vi "SubPanel_DataCollection_Rev11_v15.vi"(0 "DCPowerInformationClusterArray_Input":T4(array[cluster]), 1 "VISAPowerInfoInputArray":T3(array[cluster]), 2 "Run Data SubPanel Input":T2, 3 "RF Block Input Array":T1[](array[typedef]), 4 "Oscilloscope Info Array":T7(array[cluster]) {"vertical coupling" items=["AC", "DC", "Ground"]}, 5 "Plot Color Array":u32[](array[colorbox])=[16711686, 65351, 8978420, 14474240, 16139007, 16752640, 8958719, 16758973, 16777215, 46792, 11992992, 12961221, 16763690, 12600063, 16711835, 2953983, 40796, 13111296, 13352613, 9221011, 12964076, 12819897, 65442, 16776704, 14540253, 16740729, 10658047, 10813344, 16753521, 13413843, 8691115, 10339240, 14401205, 16746704, 7467519, 16775978, 13872558, 11387603, 13354405, 10420227, 13107364, 4060, 35208, 11817216, 7566080, 40796, 7539456, 2837073, 6372186, 7499083, 10648702, 16757152], 6 "New Run?":bool, 7 "error in":errorcluster) -> (20 "DCPowerInformationClusterArray_Output":T4(array[cluster]), 21 "VISAPowerInfoInputOutput":T3(array[cluster]), 22 "Run Data SubPanel Output":T2, 23 "RF Subpanel Output":T1[](array[typedef]), 24 "Oscilloscope Info Array":T7(array[cluster]) {"vertical coupling" items=["AC", "DC", "Ground"]}, 25 "Reinitialize?":bool, 26 "Data Was Collected?":bool, 27 "error out":errorcluster)   [LabVIEW 2019]
uses:
  Controls/DataBlockControl.ctl
  Controls/QueueDataControl_V3.ctl
  <vilib>/Utility/file.llb/Write Delimited Spreadsheet (string).vi
  <instrlib>/niScope/Acquire/Fetch/niScope Multi Fetch Binary 16.vi
  Controls/RFBlockControl.ctl
  <instrlib>/niScope/Controls/niScope vertical coupling.ctl
panel:
  in  "Total Current Y Min":dbl
  in  "Total Current Y Max":dbl
  in  "Total Voltage Y Min":dbl
  in  "Total Voltage Y Max":dbl
  in  "Total Measurement Range Update":bool
  in  "Live Measurement Range Update":bool
  in  "Live Current Y Min":dbl
  in  "Live Current Y Max":dbl
  in  "Live Voltage Y Min":dbl
  in  "Live Voltage Y Max":dbl
  out "Current Measurements Live":cluster{dbl[], dbl[]}[](graph)
  out "Voltage Measurements Live":cluster{dbl[], dbl[]}[](graph)
  out "RFSourceInfoArray":string[][](array[string])
  out "OscilloscopeInfoArray":string[][](array[string])
  out "Voltage Waveform Array":waveform(dbl)[](graph)
  out "Current Waveform Array":waveform(dbl)[](graph)
  out "DCPowerInfoArray":string[][](array[string])
  out "Current Measurements Total":cluster{dbl[], dbl[]}[](graph)
  out "Voltage Measurements Total":cluster{dbl[], dbl[]}[](graph)
  out "Exiting":bool
  out "Full Run Information":string
  out "Ready For Next Run?":bool
  in  "Next Run":bool
  out "Recording Data":bool
  in  "Record Data Toggle":bool
  out "error of collection":errorcluster
  in  "force exit SubVI":bool
  out "RF Block Parameters Output":T1
  in  "Oscilloscope Info Array":T6(array[cluster]) {"vertical coupling" items=["AC", "DC", "Ground"]}
  # "Background information (Important)\nThere are three sets of voltage/current graphs\n\nOne is live always and just shows what all the channels look like _______ Waveform Array\n\nOne is live when measuring and shows some duration of the recording _______ Measurements Live\n\nOne shows the entire duration of the run, but it will take a few seconds to compile, just be patient it will populate\n\n\nInstructions (More Important)"
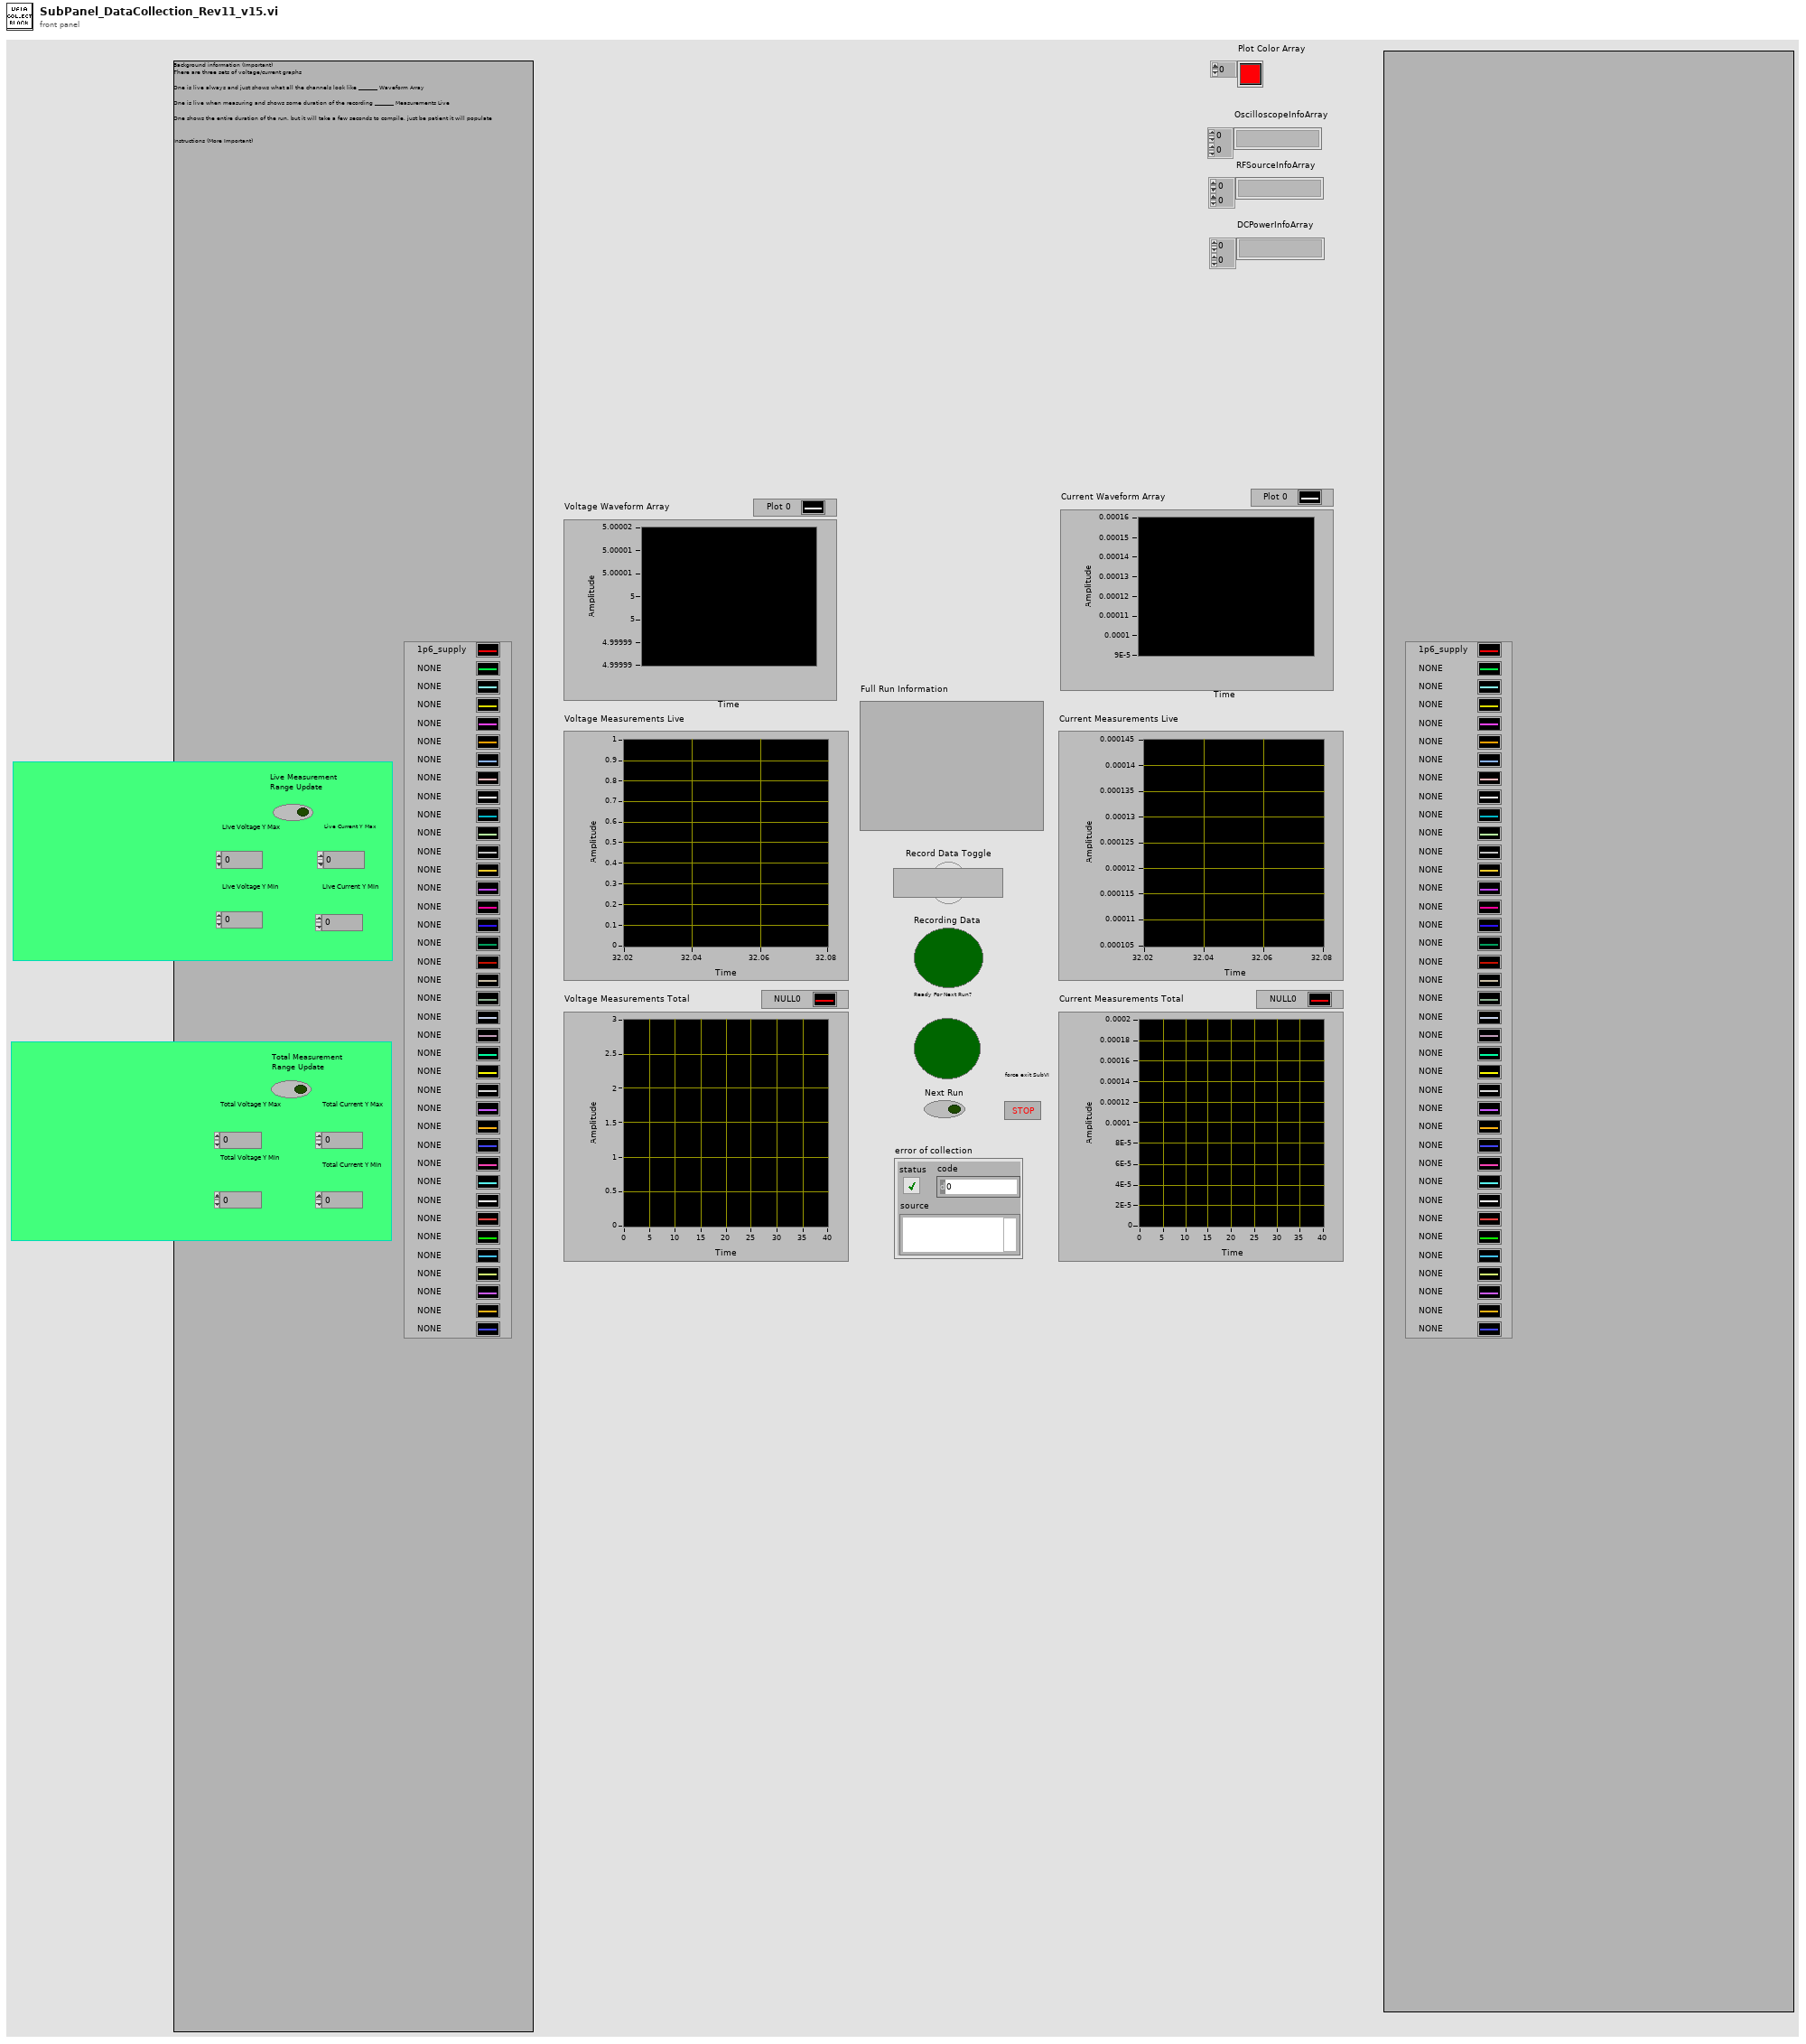
[diagram p1: front panel]
types:
  T1 = typedef "RFBlockControl.ctl" = cluster{"VISA resource name":refnum<visa-resource-name>, "RF Power State In":bool, "Frequency (GHz) Output":dbl, "Power (dBm) Output":dbl, "Instrument Name":string}
  T2 = typedef "DataBlockControl.ctl" = cluster{"Run Folder Parent Directory":path, "DUT":string, "Ion (ex Kr)":string, "Board Number":string, "Effective LET":string, "Test Type":enum16{"Single Event Latchup", "Single Event Transient", "Single Event Upset"}}
  T3 = cluster{"VISA resource name":refnum<visa-resource-name>, "String List":string, string[], "Input Array (Voltage,Current_Limit)":dbl[], "Input Array (Voltage,Current_Limit)":dbl[], "Channel Names":string[], "read buffer":string}[]
  T4 = cluster{"instrument handle out":refnum<k15>, string, string[], dbl[], string[], "Current Limit Output Array":dbl[], dbl[]}[]
  T5 = typedef "niScope vertical coupling.ctl" = i32
  T6 = cluster{"instrument handle out":refnum<k15>, "channel numbers array":string[], "channel names array":string[], "vertical range":dbl, "vertical coupling":T5, "Channel 0 50 ohms?":bool, "50 ohm vertical range (V)":dbl, "min record length":i32, "Actual Sample Rate":dbl}[]
  T7 = cluster{"instrument handle out":refnum<k15>, string[], string[], "vertical range":dbl, "vertical coupling":T5, "Channel 0 50 ohms?":bool, "50 ohm vertical range (V)":dbl, "min record length":i32, "Actual Sample Rate":dbl, "channel names list":string}[]
  T8 = typedef "QueueDataControl_V3.ctl" = cluster{"Array of fetched data":dbl[][][], "Channel Names Array":string[], "Voltage Waveform Array":waveform(dbl)[], "Current Waveform Array":waveform(dbl)[], "Resetting Time":timestamp, "Beam Logic":dbl}
  T9 = cluster{"IVI Refnum out":refnum<k15>, string, "voltage level channel 23":dbl, "Channel Name 23":string, "Current Limit":dbl, "Measure Record dt":dbl, string}[]
  T10 = cluster{timestamp[], "wfm info":cluster{"actualSamples":i32, "absoluteInitialX":dbl, "relativeInitialX":dbl, "xIncrement":dbl, "offset":dbl, "gain":dbl, "reserved1":dbl, "reserved2":dbl}[][], "wfm":i16[][][]}
  T11 = cluster{"actualSamples":i32, "absoluteInitialX":dbl, "relativeInitialX":dbl, "xIncrement":dbl, "offset":dbl, "gain":dbl, "reserved1":dbl, "reserved2":dbl}[]
  T12 = cluster{"created path array":path[], "DCPowerInformation_byChannel":cluster{"IVI Refnum out":refnum<k15>, string, "voltage level channel 23":dbl, "Channel Name 23":string, "Current Limit":dbl, "Measure Record dt":dbl, string}[], string[]}
  T13 = cluster{"Array of fetched data":dbl[][], string, i32[]}
  T14 = enum16{"open", "replace", "create", "open or create", "replace or create", "replace or create with confirmation"}
  T15 = enum16{"Single Event Latchup", "Single Event Transient", "Single Event Upset"}
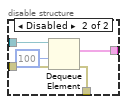
[diagram p6: hidden frame]
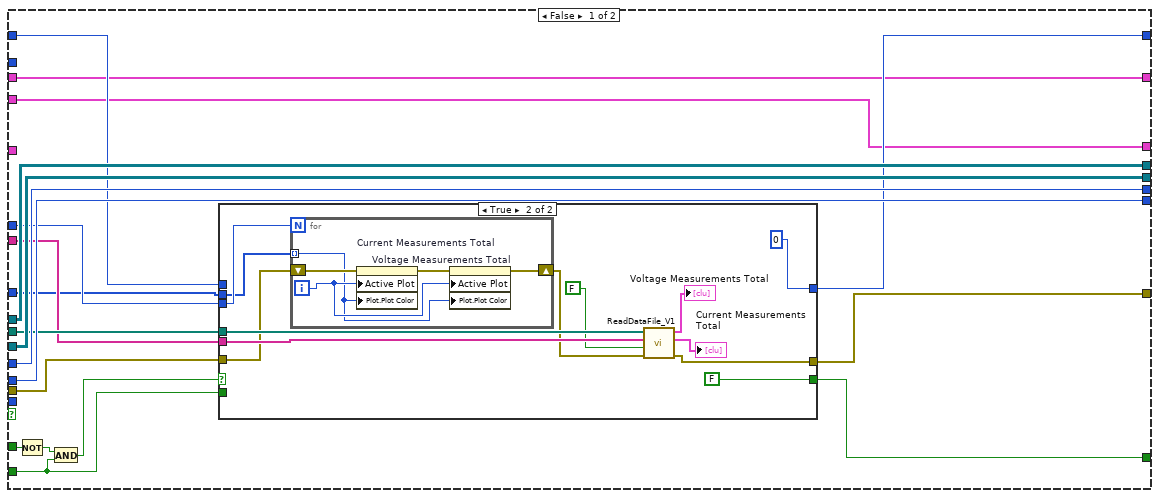
[diagram p7: hidden frame]
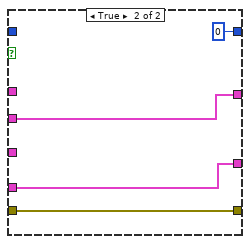
[diagram p9: hidden frame]
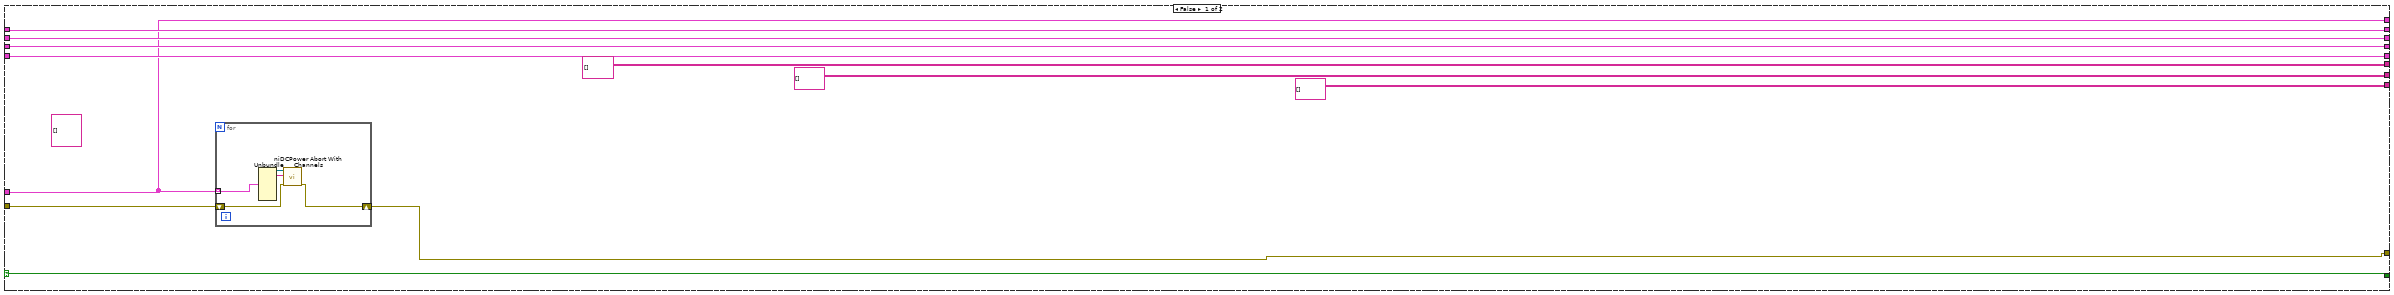
[diagram p10: hidden frame]
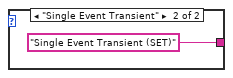
[diagram p11: hidden frame]
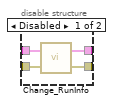
[diagram p15: hidden frame]
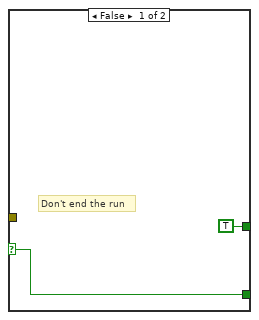
[diagram p18: hidden frame]
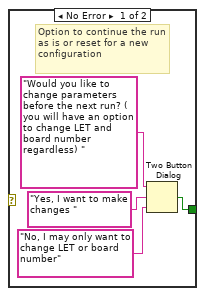
[diagram p19: hidden frame]
diagram:
  w18 = cluster{dbl[], dbl[]}[] [] ("array")
  (unwired) string[] ["Instrument Name", "Channel Name", "Instrument Channel Number", "Voltage (V)", "Current Limit (A)", "Measure Record delta Time (s)"] ("new element/subarray")
  w51 = T8 {"Array of fetched data"=[], "Channel Names Array"=[], "Voltage Waveform Array"=[], "Current Waveform Array"=[], "Resetting Time"=timestamp(0 s since 1904-01-01), "Beam Logic"=0.0} ("DCPower Queue Data Double Array Format")
  (unwired) T8 {"Array of fetched data"=[], "Channel Names Array"=[], "Voltage Waveform Array"=[], "Current Waveform Array"=[], "Resetting Time"=timestamp(0 s since 1904-01-01), "Beam Logic"=0.0} ("DCPower Double Array Queue")
  (unwired) 10000 ("binary file indexor in")
  (unwired) T2 {"Run Folder Parent Directory"=path "", "DUT"="", "Ion (ex Kr)"="", "Board Number"="", "Effective LET"="", "Test Type"=enum."Single Event Latchup"} ("Run Data Configuration")
  # "Need to make a function that will decrease the amount of loops if there are more channels active. Just exponential decay or a X/Y function but need some kind of offset which will probably be experimentally determined"
  # "Initiating the queue"
  # "echoing run information"
  # "Checking if this is a new run. If it is, a new folder is created along with references to a datafile node. If it is not new (i.e. you didn't start recording data because you needed to make a last minute change and pressed forced exit subvi), the previous folder that is theoretically empty (or just has the .txt files is used"
  # "If yes, you go into this subVI"
  # "This is the message at the beginning confirming if you want to make small changes to the program (i.e. LET)"
  # "Parameters from the configuration stage of this program"
  # "Reset the graph that is saving every 10 seconds of data. Every reset the low bound of the ten seconds is"
  # "Need to change to reflect number of channels that are being recorded. Collect this from a parameters file eventually that will be created"
  # "Indicator if the system is ready for another run. Also indicates if data was actually collected"
  # "Resets the system to start recording"
  # "A flag to ensure the warning message shows only once and doesn't lock the system"
  # "Initiating all of the DC Power instruments (doing this here so because we force abort channels in the DCPower setup because buffer overflow issues. Iterating over the instrument array and the active channel list"
  n1 = flat-sequence {
    tunnel: [w90] -> w67
    tunnel: "error in" -> [w80]
    tunnel: [w94] -> w72
    tunnel: "Run Data SubPanel Input" -> [w82]
    frame #0 {
      n2 = disable-structure shown="Enabled" {
        disable-tunnel: w80 -> [w97 w108]
        disable-tunnel: [w106 w108] -> w79
        frame Enabled {
          n3 = property on="Voltage Measurements Live" class="XYGraph (strict)"(error in=w97, "BG Color"=u32 0 ("Plot.Plot Color"), "Plot.Plot Interpolation"=u8 2) -> (error out=w96:errorcluster)  [unwired: 1 in, 1 out]
          n4 = property on="Current Measurements Live" class="XYGraph (strict)"(error in=w96, "BG Color"=u32 0 ("Plot.Plot Color"), "Plot.Plot Interpolation"=u8 2) -> (error out=w95:errorcluster)  [unwired: 1 in, 1 out]
          n5 = property on="Voltage Measurements Total" class="XYGraph (strict)"(error in=w95, "BG Color"=u32 0 ("Plot.Plot Color"), "Plot.Plot Interpolation"=u8 2) -> (error out=w107:errorcluster)  [unwired: 1 in, 1 out]
          n6 = property on="Current Measurements Total" class="XYGraph (strict)"(error in=w107, "BG Color"=u32 0 ("Plot.Plot Color"), "Plot.Plot Interpolation"=u8 2) -> (error out=w106:errorcluster)  [unwired: 1 in, 1 out]
        }
        frame Disabled {
        }
      }
      n7 = local write "Voltage Measurements Total"(cluster{dbl[], dbl[]}[] [] ("Voltage Measurements")) -> ()
      n8 = local write "Current Measurements Total"(cluster{dbl[], dbl[]}[] [] ("Current Measurements")) -> ()
      n9 = local write "Recording Data"(FALSE ("Recording Data")) -> ()
      n10 = local write "Exiting"(FALSE ("Forced Exit")) -> ()
      n11 = call "Convert_RunInfoCluster_2_RunInfoStringList.vi"("error in"=w79, "Run Number"="", "Run Data SubPanel Input"=w82) -> ("error output"=w83:errorcluster, "Run Data Output"=w84:string)
      n12 = call "Display Message to User"("error in (no error)"=w83, "Enable"=TRUE, "Message"=w84) -> ("error out"=w90:errorcluster)  [unwired: 7 in, 1 out]
      n13 = Two Button Dialog(message="Changing the LET?", 1:"No" ("F button name (\"Cancel\")"), 2:"Yes" ("T button name (\"OK\")")) -> (T button?=w94:bool)
    }
  }
  n14 = call "Convert_InstrumentReferenceArray_2_ChannelReferenceArray.vi"("error in (no error)"=w67, "DCPowerInformationClusterArray_Input"="DCPowerInformationClusterArray_Input") -> ("error out"=w66:errorcluster, "DCPowerInformation_byChannel"=w12:T9)
  n15 = case shown="True" w72 {
    tunnel: "Run Data SubPanel Input" -> [w110 w114]
    tunnel: [w110 w113] -> w26
    tunnel: [w109 w112] -> w68
    tunnel: w66 -> [w109 w111]
    frame False {
    }
    frame True {
      n16 = disable-structure shown="Enabled" {
        disable-tunnel: w114 -> [w118 w120]
        disable-tunnel: [w117 w119] -> w113
        disable-tunnel: [w116 w122] -> w112
        disable-tunnel: w111 -> [w115 w121]
        frame Disabled {
          n17 = call "Change_RunInfo.vi"("error in (no error)"=w115, "Run Data SubPanel in"=w118) -> ("error out"=w116:errorcluster, "Run Data SubPanel out"=w117:T2)
        }
        frame Enabled {
          n18 = call "Change_RunInfo_V2.vi"("error in (no error)"=w121, "Run Data SubPanel in"=w120) -> ("error out"=w122:errorcluster, "Run Data SubPanel out"=w119:T2)
        }
      }
    }
  }
  n19 = Unbundle(w26) -> ("Run Folder Parent Directory"=w69:path)  [unwired: 5 out]
  n20 = List Folder(path=w69, error in=w68) -> (folder names=w70:string[], error out=w54:errorcluster)  [unwired: 2 in, 2 out]
  n21 = Array Size(array=w70) -> (size(s)=w57:i32)
  n22 = case shown="True" "New Run?" {
    selector: "New Run?" -> [w124 w127]
    tunnel: [w125 w129] -> w58
    tunnel: w57 -> [w125 w128]
    tunnel: [w124 w127] -> w56
    tunnel: [w123 w126] -> w55
    tunnel: w54 -> [w123 w126]
    frame False {
    }
    frame True {
      n23 = Increment(x=w128) -> (x+1=w129:i32)
    }
  }
  n24 = Number To Decimal String(number=w58) -> (decimal integer string=w61:string)  [unwired: 1 in]
  n25 = Concatenate Strings("Run_", w61) -> (w25:string)
  n26 = Array Size(array=w12) -> (size(s)=w53:i32)
  n27 = call "InitialFileFolderCreation_V2.vi"("New Run?"=w56, "error in (no error)"=w55, "Run Number"=w25, "Subfolders&NumChannelsRecorded"=w53, "base path"=w69) -> ("error out"=w24:errorcluster, "SupplementalDataFileReferenceObjectArrayWsubfolders"=w64:refnum<file>[][], "DataFileReferenceObjectArrayWsubfolders"=w65:refnum<file>[][], "created path array"=w30:path[])  [unwired: 3 in]
  n28 = call "Convert_RunInfoCluster_2_RunInfoStringList.vi"("error in"=w24, "Run Number"=w25, "Run Data SubPanel Input"=w26) -> ("error output"=w23:errorcluster, "Run Data Output"=→"Full Run Information":string)
  n29 = for {
    shift-right: [w130] -> w9
    shift-left: w23 -> [w132]
    tunnel: "DCPowerInformationClusterArray_Input" -> [w134] mode=indexing
    n30 = Unbundle(w134) -> ("instrument handle out"=w131:refnum<k15>, w133:string)  [unwired: 5 out]
    n31 = call <instrlib>:"niDCPower Initiate With Channels.vi"("error in (no error)"=w132, "channel name"=w133, "instrument handle"=w131) -> ("error out"=w130:errorcluster)  [unwired: 7 in, 1 out]
  }
  n32 = for {
    shift-right: [w137] -> w10
    shift-left: w9 -> [w139]
    tunnel: "Plot Color Array" -> [_] mode=indexing
    i -> [w135]
    w136 = "NONE" ("Plot.Plot Name")
    n33 = property on="Current Measurements Live" class="XYGraph (strict)"(error in=w139, "Active Plot"=w135, "Plot.Plot Name"=w136) -> (error out=w138:errorcluster)  [unwired: 1 in, 1 out]
    n34 = property on="Voltage Measurements Live" class="XYGraph (strict)"(error in=w138, "Active Plot"=w135, "Plot.Plot Name"=w136) -> (error out=w137:errorcluster)  [unwired: 1 in, 1 out]
  }
  n35 = case shown="Error .." w10 {
    selector: w10 -> [w140 _]
    tunnel: [w140 w141] -> w4
    tunnel: w9 -> [_ w141]
    frame No Error {
    }
    frame Error {
    }
  }
  n36 = for {
    tunnel: w12 -> [w144] mode=indexing
    tunnel: [w147] -> w13 mode=indexing
    shift-right: [w143] -> w14
    shift-left: w4 -> [w146]
    tunnel: "Plot Color Array" -> [w142] mode=indexing
    i -> [w148]
    # "Creating Array of Channel Names"
    n37 = Unbundle(w144) -> ("Channel Name 23"=w147:string)  [unwired: 6 out]
    n38 = property on="Current Measurements Live" class="XYGraph (strict)"(error in=w146, "Active Plot"=w148, "Plot.Plot Name"=w147, "Plot.Plot Color"=w142) -> (error out=w145:errorcluster)  [unwired: 1 in, 1 out]
    n39 = property on="Voltage Measurements Live" class="XYGraph (strict)"(error in=w145, "Active Plot"=w148, "Plot.Plot Name"=w147, "Plot.Plot Color"=w142) -> (error out=w143:errorcluster)  [unwired: 1 in, 1 out]
  }
  n40 = disable-structure shown="Enabled" {
    disable-tunnel: w14 -> [w152 w154]
    disable-tunnel: [w151 w154] -> w3
    disable-tunnel: [w150 _] -> w15
    disable-tunnel: w51 -> [w149 _]
    frame Enabled {
      n41 = Obtain Queue(name (unnamed)="DCPowerQueue", element data type=w149, error in (no error)=w152) -> (queue out=w150:refnum<queue>, error out=w151:errorcluster)  [unwired: 2 in, 1 out]
    }
    frame Disabled {
    }
  }
  n42 = disable-structure shown="Disabled" {
    disable-tunnel: "Oscilloscope Info Array" -> [w160 _]
    disable-tunnel: w3 -> [w159 _]
    frame Disabled {
      w155 = T10 {[], "wfm info"=[], "wfm"=[]} ("output cluster")
      n43 = Obtain Queue(name (unnamed)="OscilloscopeDataQueue", element data type=w155, error in (no error)=w159) -> (queue out=w156:refnum<queue>, error out=w158:errorcluster)  [unwired: 2 in, 1 out]
      n44 = Unbundle() -> ()  [unwired: 1 in, 2 out]
      n45 = while {
        shift-right: _ -> [_]
        shift-left: w158 -> [w169]
        shift-right: [w164] -> _
        shift-left: w160 -> [w164]
        tunnel: w156 -> [w167]
        tunnel: w155 -> [w166]
        stop <- _ stop-if-true
        # "BASE OFF OF TAMU POWER SCRIPTS"
        n46 = for {
          tunnel: w164 -> [w188] mode=indexing
          shift-right: [w182] -> w165
          shift-left: w169 -> [w183]
          tunnel: [w181] -> w162 mode=indexing
          tunnel: [w180] -> w161 mode=indexing
          tunnel: [w179] -> w163 mode=indexing
          n47 = Unbundle By Name(w188) -> ("instrument handle out"=w187:refnum<k15>, "channel names list"=w185:string)
          n48 = Get Date/Time In Seconds() -> (seconds since 1Jan1904=w179:timestamp)
          n49 = call-poly <instrlib>:"niScope Fetch (poly).vi"("timeout"=0.0, "error in"=w183, "numSamples"=-1, "channels"=w185, "instrument handle"=w187) -> ("error out"=w182:errorcluster, "wfm"=w180:i16[][], "wfm info"=w181:T11)  [unwired: 3 in, 1 out]
        }
        n50 = Bundle(cluster=w166, w163, "wfm info"=w162, "wfm"=w161) -> (w168:T10)
        n51 = for {
          tunnel: w163 -> [w171] mode=indexing
          tunnel: w162 -> [w175]
          tunnel: w161 -> [w174]
          i -> [w173]
          n52 = Index Array(array=w175, index (col)=w173) -> (element=w172:T11)  [unwired: 1 in]
          n53 = Index Array(array=w174, index (dim 0)=w173) -> (element=w170:i16[][])  [unwired: 2 in]
          n54 = for {
            tunnel: w172 -> [w178] mode=indexing
            tunnel: w171 -> [w177]
            tunnel: w170 -> [_] mode=indexing
            n55 = Unbundle(w178) -> ("xIncrement"=w176:dbl)  [unwired: 7 out]
            n56 = Bundle By Name("dt"=w176, "t0"=w177) -> ()  [unwired: 2 in, 1 out]
          }
        }
        n57 = Enqueue Element(queue=w167, element=w168, error in (no error)=w165) -> ()  [unwired: 1 in, 3 out]
      }
      n58 = while {
        stop <- _ stop-if-true
      }
    }
    frame Enabled {
    }
  }
  n59 = Bundle("created path array"=w30, "DCPowerInformation_byChannel"=w12, w13) -> (w43:T12)  [unwired: 1 in]
  n60 = Array Size(array=w13) -> (size(s)=w17:i32)
  n61 = Get Date/Time In Seconds() -> (seconds since 1Jan1904=w28:timestamp)
  n62 = while {
    tunnel: w15 -> [w228]
    shift-right: [w189] -> w48
    shift-left: w3 -> [w227]
    tunnel: w30 -> [w224]
    shift-right: [w217] -> w50
    shift-left: w65 -> [w225]
    shift-right: [w216] -> w49
    shift-left: w64 -> [w223]
    shift-right: [w219] -> _
    shift-left: 0 ("binary file indexor in") -> [w222]
    shift-right: [w218] -> _
    shift-left: 0 ("binary file indexor in") -> [w221]
    tunnel: 1000 ("binary file indexor in") -> [w220]
    tunnel: w13 -> [w226]
    tunnel: w17 -> [w195]
    shift-right: [w205] -> _
    shift-left: FALSE -> [w204]
    shift-right: [w201] -> _
    shift-left: 0 -> [w202]
    shift-right: [w200] -> _
    shift-left: w18 -> [w197]
    shift-right: [w199] -> _
    shift-left: w18 -> [w198]
    tunnel: 251 ("y") -> [w196]
    tunnel: "Plot Color Array" -> [w194]
    stop <- w213 stop-if-true
    # "If recording data is on, there should always be elements in the queue, so I shouldn't have to worry about a state where the \"recording data\" is active but there is no data in the queue, if so, then I'll just have to find an alternative to the OR statement"
    n63 = Get Queue Status(queue=w228, error in (no error)=w227) -> (queue out=w210:refnum<queue>, error out=w211:errorcluster, # elements in queue=w206:i32)  [unwired: 1 in, 5 out]
    n64 = local read "Recording Data"() -> (w203:bool)
    n65 = disable-structure shown="Enabled" {
      disable-tunnel: [w248 w250] -> w212
      disable-tunnel: w211 -> [w247 w252]
      disable-tunnel: w210 -> [w246 w253]
      disable-tunnel: [w245 w249] -> w209
      frame Enabled {
        n66 = Flush Queue(queue=w246, error in (no error)=w247) -> (remaining elements=w245:T8[], error out=w248:errorcluster)  [unwired: 1 out]
      }
      frame Disabled {
        n67 = Dequeue Element(queue=w253, timeout in ms (-1)=100, error in (no error)=w252) -> (element=w249:T8, error out=w250:errorcluster)  [unwired: 2 out]
      }
    }
    n68 = Not Equal To 0?(x=w206) -> (x != 0?=w208:bool)
    n69 = And(x=w208, y=w203) -> (x .and. y?=w207:bool)
    n70 = case shown="True" w207 {
      tunnel: w209 -> [_ w325]
      tunnel: w212 -> [w263 w319]
      tunnel: w226 -> [w264 w312]
      tunnel: w225 -> [w271 w324]
      tunnel: w224 -> [w265 w323]
      tunnel: w223 -> [w272 w322]
      tunnel: w222 -> [w270 w321]
      tunnel: w221 -> [w269 w311]
      tunnel: w220 -> [_ w310]
      tunnel: [w270 w318] -> w219
      tunnel: [w269 w317] -> w218
      tunnel: [w271 w314] -> w217
      tunnel: [w272 w313] -> w216
      tunnel: [w262 w304] -> w193
      tunnel: [w261 TRUE] -> w205
      tunnel: w204 -> [w260 _]
      tunnel: w203 -> [w268 _]
      tunnel: w202 -> [w259 w302]
      tunnel: [w258 w301] -> w201
      tunnel: [w257 w308] -> w200
      tunnel: [w256 w305] -> w199
      tunnel: w198 -> [w256 w300]
      tunnel: w197 -> [w257 w299]
      tunnel: w196 -> [_ w293]
      tunnel: w195 -> [w255 _]
      tunnel: w194 -> [w254 _]
      frame False {
        n71 = Not(x=w268) -> (.not. x?=w267:bool)
        n72 = And(x=w267, y=w260) -> (x .and. y?=w266:bool)
        n73 = case shown="True" w266 {
          tunnel: w265 -> [_ w287]
          tunnel: w264 -> [_ w286]
          tunnel: w263 -> [w275 w279]
          tunnel: [w275 w284] -> w262
          tunnel: [w274 FALSE] -> w261
          tunnel: w260 -> [w274 _]
          tunnel: w259 -> [w273 _]
          tunnel: [w273 0] -> w258
          tunnel: w255 -> [_ w277]
          tunnel: w254 -> [_ w276]
          frame False {
          }
          frame True {
            n74 = for {
              N: w277 -> [_]
              shift-right: [w290] -> w278
              shift-left: w279 -> [w291]
              tunnel: w276 -> [w288] mode=indexing
              i -> [w289]
              n75 = property on="Current Measurements Total" class="XYGraph (strict)"(error in=w291, "Active Plot"=w289, "Plot.Plot Color"=w288) -> (error out=w292:errorcluster)  [unwired: 1 in, 1 out]
              n76 = property on="Voltage Measurements Total" class="XYGraph (strict)"(error in=w292, "Active Plot"=w289, "Plot.Plot Color"=w288) -> (error out=w290:errorcluster)  [unwired: 1 in, 1 out]
            }
            n77 = call "ReadDataFile_V1.vi"("error in (no error)"=w278, "Create CSV files?"=FALSE, "Channel Names Array"=w286, "DataFolder Path"=w287) -> ("error out"=w284:errorcluster, "Current Measurements"=→"Current Measurements Total":cluster{dbl[], dbl[]}[], "Voltage Measurements"=→"Voltage Measurements Total":cluster{dbl[], dbl[]}[])  [unwired: 5 in]
          }
        }
      }
      frame True {
        # "structure where each channel has its own data and supplemental file. Intent for faster data reading speeds in post processing. Probably not since would be i^3, but if we used multiple cores, maybe it would be advantageous"
        n78 = call "FilePathCreation_DCPower_V2.vi"("binary file input reference array 1"=w324, "Channel Name Input array"=w312, "data output directory folder"=w323, "binary file indexor in"=w321, "Reset counter in"=w311, "error in (no error)"=w319, "binary file input reference array 2"=w322, "reset threshold"=w310) -> ("binary file output reference array"=w316:refnum<file>[], "binary file output reference array 2"=w315:refnum<file>[], "binary file indexor out"=w318:i32, "reset counter out"=w317:i32, "error out"=w320:errorcluster)  [unwired: 3 in]
        n79 = for {
          shift-right: [w372] -> w303
          shift-left: w320 -> [w373]
          tunnel: w325 -> [w382]
          tunnel: w315 -> [w379] mode=indexing
          tunnel: w316 -> [w378] mode=indexing
          tunnel: [w377] -> w313 mode=indexing
          tunnel: [w371] -> w314 mode=indexing
          tunnel: [w360] -> w307 mode=indexing
          tunnel: [w359] -> w306 mode=indexing
          i -> [w376]
          n80 = for {
            tunnel: w382 -> [w395] mode=indexing
            tunnel: w376 -> [w392]
            tunnel: [w387] -> w367 mode=concatenating
            tunnel: [w391] -> w381
            tunnel: w379 -> [w390]
            tunnel: w378 -> [w388]
            tunnel: [w388] -> w374
            tunnel: [w390] -> w377
            tunnel: [w389] -> w380 mode=concatenating
            n81 = Unbundle(w395) -> ("Array of fetched data"=w394:dbl[][][], "Channel Names Array"=w393:string[])  [unwired: 4 out]
            n82 = Index Array(array=w393, index=w392) -> (element=w391:string)
            n83 = Index Array(array=w394, index (dim 0)=w392) -> (element=w387:dbl[][])  [unwired: 2 in]
            n84 = Array Size(array=w387) -> (size(s)=w389:i32[])
          }
          n85 = Bundle("Array of fetched data"=w367, w381, w380) -> (w375:T13)  [unwired: 1 in]
          n86 = Index Array(array=w367, index (row)=2) -> (element=w364:dbl[])  [unwired: 1 in]
          n87 = Index Array(array=w367, index (row)=1) -> (element=w365:dbl[])  [unwired: 1 in]
          n88 = Index Array(array=w367, index (row)=0) -> (element=w366:dbl[])  [unwired: 1 in]
          n89 = call "DataFileNode_Entry_V4.vi"("error in (no error)"=w373, "Queued Elements"=w375, "Byte Stream File in"=w374) -> ("error out"=w372:errorcluster, "Byte Stream File out"=w371:refnum<file>)  [unwired: 7 in]
          n90 = for {
            tunnel: [w384] -> w363 mode=indexing if=w383
            tunnel: w366 -> [w384] mode=indexing
            tunnel: [w386] -> w361 mode=indexing if=w383
            tunnel: w365 -> [w386] mode=indexing
            tunnel: [w385] -> w362 mode=indexing if=w383
            tunnel: w364 -> [w385] mode=indexing
            n91 = Not Equal To 0?(x=w384) -> (x != 0?=w383:bool)
          }
          n92 = Bundle(w363, w361) -> (w360:cluster{dbl[], dbl[]})  [unwired: 1 in]
          n93 = Bundle(w363, w362) -> (w359:cluster{dbl[], dbl[]})  [unwired: 1 in]
        }
        n94 = Greater?(x=w302, y=w293) -> (0:w295:bool)
        n95 = Array Size(array=w299) -> (size(s)=w298:i32)
        n96 = Equal?(x=w298, y=0) -> (x = y?=w296:bool)
        n97 = Or(x=w295, y=w296) -> (x .or. y?=w294:bool)
        n98 = case shown="False" w294 {
          tunnel: [w331 w355] -> w308
          tunnel: w299 -> [w335 _]
          tunnel: w307 -> [w334 w355]
          tunnel: w300 -> [w333 _]
          tunnel: w306 -> [w332 w356]
          tunnel: [w330 w356] -> w305
          tunnel: [w329 w358] -> w304
          tunnel: w303 -> [w328 w358]
          tunnel: w302 -> [w327 _]
          tunnel: [w326 0] -> w301
          frame False {
            n99 = for {
              tunnel: w335 -> [w354] mode=indexing
              tunnel: w334 -> [w351] mode=indexing
              tunnel: w333 -> [w348] mode=indexing
              tunnel: w332 -> [w347] mode=indexing
              tunnel: [w338] -> w331 mode=indexing
              tunnel: [w337] -> w330 mode=indexing
              shift-right: [w336] -> w329
              shift-left: w328 -> [w336]
              n100 = Unbundle(w354) -> (w353:dbl[], w352:dbl[])
              n101 = Unbundle(w351) -> (w350:dbl[], w349:dbl[])
              n102 = Unbundle(w348) -> (w346:dbl[], w345:dbl[])
              n103 = Unbundle(w347) -> (w344:dbl[], w343:dbl[])
              n104 = Insert Into Array(array=w346, new element=w344) -> (w341:dbl[])  [unwired: 1 in]
              n105 = Insert Into Array(array=w353, new element=w350) -> (w339:dbl[])  [unwired: 1 in]
              n106 = Insert Into Array(array=w345, new element=w343) -> (w342:dbl[])  [unwired: 1 in]
              n107 = Insert Into Array(array=w352, new element=w349) -> (w340:dbl[])  [unwired: 1 in]
              n108 = Bundle(w341, w342) -> (w337:cluster{dbl[], dbl[]})  [unwired: 1 in]
              n109 = Bundle(w339, w340) -> (w338:cluster{dbl[], dbl[]})  [unwired: 1 in]
            }
            n110 = Increment(x=w327) -> (x+1=w326:i32)
          }
          frame True {
          }
        }
        "Voltage Measurements Live" <- w308
        "Current Measurements Live" <- w305
      }
    }
    n111 = local read "Exiting"() -> (w215:bool)
    n112 = Equal To 0?(x=w206) -> (x = 0?=w214:bool)
    n113 = case shown="True" "Live Measurement Range Update" {
      tunnel: w193 -> [w237 w244]
      tunnel: [w237 w242] -> w190
      frame False {
      }
      frame True {
        n114 = property on="Voltage Measurements Live" class="XYGraph (strict)"(error in=w244, "YScale.Maximum"="Live Voltage Y Max", "YScale.Minimum"="Live Voltage Y Min") -> (error out=w243:errorcluster)  [unwired: 1 in, 1 out]
        n115 = property on="Current Measurements Live" class="XYGraph (strict)"(error in=w243, "YScale.Maximum"="Live Current Y Max", "YScale.Minimum"="Live Current Y Min") -> (error out=w242:errorcluster)  [unwired: 1 in, 1 out]
      }
    }
    n116 = And(x=w214, y=w215) -> (x .and. y?=w213:bool)
    n117 = case shown="True" "Total Measurement Range Update" {
      tunnel: w190 -> [w229 w236]
      tunnel: [w229 w234] -> w189
      frame False {
      }
      frame True {
        n118 = property on="Voltage Measurements Total" class="XYGraph (strict)"(error in=w236, "YScale.Maximum"="Total Voltage Y Max", "YScale.Minimum"="Total Voltage Y Min") -> (error out=w235:errorcluster)  [unwired: 1 in, 1 out]
        n119 = property on="Current Measurements Total" class="XYGraph (strict)"(error in=w235, "YScale.Maximum"="Total Current Y Max", "YScale.Minimum"="Total Current Y Min") -> (error out=w234:errorcluster)  [unwired: 1 in, 1 out]
      }
    }
  }
  n120 = while {
    shift-right: [w426] -> w34
    shift-left: "DCPowerInformationClusterArray_Input" -> [w426]
    shift-right: [w430] -> w36
    shift-left: "VISAPowerInfoInputArray" -> [w430]
    shift-right: [w429] -> w38
    shift-left: w26 -> [w429]
    shift-right: [w428] -> w40
    shift-left: "RF Block Input Array" -> [w428]
    shift-right: [w427] -> w42
    shift-left: "Oscilloscope Info Array" -> [w427]
    shift-right: [w396] -> w52
    shift-left: w3 -> [w424]
    tunnel: w12 -> [w425]
    shift-right: [w423] -> _
    shift-left: FALSE -> [w420]
    tunnel: w15 -> [w422]
    shift-right: [w406] -> _
    shift-left: FALSE -> [w411]
    tunnel: [w415] -> w76
    shift-right: [w409] -> _
    shift-left: TRUE ("x .and. y?") -> [w410]
    shift-right: [w407] -> _
    shift-left: w28 -> [w408]
    tunnel: [w406] -> w33
    tunnel: w51 -> [w404]
    shift-right: [w401] -> w6
    shift-left: timestamp(0 s since 1904-01-01) ("seconds since 1Jan1904") -> [w400]
    stop <- w405 stop-if-true
    # "If I am going to reset the entire configuration or if we are going up in LET only. True, reset the system. False, don't reset the system"
    n121 = Not(x=w411) -> (.not. x?=w413:bool)
    n122 = And(x="Record Data Toggle", y=w413) -> (x .and. y?=w414:bool)
    "Recording Data" <- w414
    n123 = case shown="True" w414 {
      tunnel: w425 -> [w459 w474]
      tunnel: w424 -> [w457 w481]
      tunnel: [w447 w469] -> w403
      tunnel: [w448 w468] -> w402
      tunnel: w420 -> [_ w479]
      tunnel: [FALSE w480] -> w423
      tunnel: w422 -> [_ w478]
      tunnel: [w446 w477] -> w418
      tunnel: "Record Data Toggle" -> [w454 _]
      tunnel: w411 -> [w455 _]
      tunnel: w410 -> [w450 _]
      tunnel: [w451 TRUE] -> w409
      tunnel: w408 -> [w449 w482]
      tunnel: [w449 w472] -> w407
      tunnel: w404 -> [_ w476]
      tunnel: [w445 w466] -> w401
      tunnel: w400 -> [w445 w465]
      frame False {
        n124 = And(x=w454, y=w455) -> (x .and. y?=w453:bool)
        n125 = And(x=w450, y=w453) -> (x .and. y?=w452:bool)
        n126 = case shown="True" w452 {
          tunnel: [w461 w463] -> w456
          tunnel: w457 -> [w461 w464]
          tunnel: [w460 FALSE] -> w451
          tunnel: w450 -> [w460 _]
          frame False {
          }
          frame True {
            n127 = call "Display Message to User2"("error in (no error)"=w464) -> ("error out"=w463:errorcluster)  [unwired: 9 in, 1 out]
          }
        }
        n128 = call "Fetch&Process_Measurements_V4.vi"("DCPowerInformation_byChannel"=w459, "Initial Time"=w449, "error in (no error)"=w456) -> ("Current Waveform Array"=w447:waveform(dbl)[], "Voltage Waveform Array"=w448:waveform(dbl)[], "error out"=w446:errorcluster)  [unwired: 6 in, 4 out]
      }
      frame True {
        n129 = case shown="True" w479 {
          tunnel: [w484 w490] -> w472
          tunnel: w482 -> [_ w490]
          tunnel: w481 -> [w485 w489]
          tunnel: [w485 w489] -> w473
          tunnel: [TRUE w488] -> w480
          tunnel: w479 -> [_ w488]
          tunnel: [w484 w487] -> w466
          tunnel: w465 -> [_ w487]
          frame False {
            n130 = Get Date/Time In Seconds() -> (seconds since 1Jan1904=w484:timestamp)
          }
          frame True {
          }
        }
        n131 = call "Fetch&Process_Measurements_V4.vi"("DCPowerInformation_byChannel"=w474, "Initial Time"=w472, "error in (no error)"=w473) -> ("Data As dbl Array"=w471:dbl[][][], "Channel Number Array"=w470:string[], "Current Waveform Array"=w469:waveform(dbl)[], "Voltage Waveform Array"=w468:waveform(dbl)[], "error out"=w467:errorcluster)  [unwired: 6 in, 2 out]
        n132 = Bundle(cluster=w476, "Array of fetched data"=w471, "Channel Names Array"=w470) -> (w475:T8)  [unwired: 4 in]
        n133 = Enqueue Element(queue=w478, element=w475, error in (no error)=w467) -> (error out=w477:errorcluster)  [unwired: 1 in, 2 out]
      }
    }
    "Current Waveform Array" <- w403
    "Voltage Waveform Array" <- w402
    n134 = Not(x=w414) -> (.not. x?=w421:bool)
    n135 = And(x=w421, y=w420) -> (x .and. y?=w419:bool)
    n136 = case shown="True" w419 {
      tunnel: w418 -> [w441 w443]
      tunnel: [w442 TRUE] -> w406
      tunnel: w411 -> [w442 _]
      tunnel: [w441 w443] -> w396
      frame False {
      }
      frame True {
      }
    }
    "error of collection" <- w396
    "Ready For Next Run?" <- w406
    n137 = And(x="Next Run", y=w406) -> (x .and. y?=w417:bool)
    n138 = Or(x="force exit SubVI", y=w417) -> (x .or. y?=w398:bool)
    n139 = Or(x=w396, y=w398) -> (x .or. y?=w397:bool)
    n140 = case shown="True" w397 {
      selector: w397 -> [w432 _]
      tunnel: w396 -> [_ w435]
      tunnel: [w432 TRUE] -> w405
      tunnel: [TRUE ("T button?") w433] -> w415
      frame False {
        # "Don't end the run"
      }
      frame True {
        n141 = case shown="Error .." w435 {
          tunnel: [w436 TRUE] -> w433
          frame No Error {
            # "Option to continue the run as is or reset for a new configuration"
            n142 = Two Button Dialog(message="Would you like to change parameters before the next run? ( you will have an option to change LET and board number regardless) ", 1:"No, I may only want to change LET or board number" ("F button name (\"Cancel\")"), 2:"Yes, I want to make changes " ("T button name (\"OK\")")) -> (T button?=w436:bool)
          }
          frame Error {
            # "End the run immediately. There is an error or an immediate issue with the VI"
          }
        }
      }
    }
    "Exiting" <- w405
  }
  "Reinitialize?" <- w76
  n143 = for {
    tunnel: w50 -> [w495] mode=indexing
    tunnel: w49 -> [w493] mode=indexing
    shift-right: [w491] -> w47
    shift-left: w48 -> [w494]
    n144 = Close File(refnum=w495, error in=w494) -> (error out=w492:errorcluster)  [unwired: 1 out]
    n145 = Close File(refnum=w493, error in=w492) -> (error out=w491:errorcluster)  [unwired: 1 out]
  }
  n146 = Merge Errors(w52, w47) -> (w44:errorcluster)
  n147 = Unbundle(w43) -> ("created path array"=w8:path[])  [unwired: 2 out]
  n148 = case shown="True" w33 {
    selector: w33 -> [w502 w642]
    tunnel: w44 -> [w497 w648]
    tunnel: [w506 w580] -> w1
    tunnel: w42 -> [w506 w647]
    tunnel: [w505 w582] -> w41
    tunnel: w40 -> [w505 w646]
    tunnel: [w504 w568] -> w39
    tunnel: w38 -> [w504 w645]
    tunnel: [w503 w585] -> w37
    tunnel: w36 -> [w503 w644]
    tunnel: [w498 w587] -> w35
    tunnel: w34 -> [w498 w643]
    tunnel: [w502 w642] -> w32
    tunnel: [string[][] [] ("DCPowerInfoArray") w578] -> w31
    tunnel: w8 -> [_ w513]
    tunnel: [string[][] [] ("DCPowerInfoArray") w576] -> w2
    tunnel: [string[][] [] ("DCPowerInfoArray") w570] -> w20
    tunnel: [w496 w515] -> w7
    tunnel: w6 -> [_ w514]
    frame False {
      (unwired) string[][][] []
      n149 = for {
        tunnel: w498 -> [w509] mode=indexing
        shift-right: [w510] -> w496
        shift-left: w497 -> [w511]
        n150 = Unbundle(w509) -> ("instrument handle out"=w508:refnum<k15>, w507:string)  [unwired: 5 out]
        n151 = call <instrlib>:"niDCPower Abort With Channels.vi"("error in (no error)"=w511, "channel name"=w507, "instrument handle"=w508) -> ("error out"=w510:errorcluster)  [unwired: 7 in, 1 out]
      }
    }
    frame True {
      # "This will be indexed eventually"
      n152 = for {
        shift-right: [w741] -> w512
        shift-left: w648 -> [w753]
        tunnel: w643 -> [w744] mode=indexing
        shift-right: [w752] -> w618
        shift-left: w647 -> [w752]
        shift-right: [w751] -> w617
        shift-left: w646 -> [w751]
        shift-right: [w750] -> w616
        shift-left: w645 -> [w750]
        shift-right: [w749] -> w615
        shift-left: w644 -> [w749]
        shift-right: [w748] -> w614
        shift-left: w643 -> [w748]
        shift-right: [w746] -> w619
        shift-left: string[][] [] ("DCPowerInfoArray") -> [w747]
        # "This puts all the instruments together in one output"
        n153 = Unbundle(w744) -> ("instrument handle out"=w755:refnum<k15>, w754:string)  [unwired: 5 out]
        n154 = call <instrlib>:"niDCPower Abort With Channels.vi"("error in (no error)"=w753, "channel name"=w754, "instrument handle"=w755) -> ("error out"=w742:errorcluster)  [unwired: 7 in, 1 out]
        n155 = call "DCPower_ParameterCreation.vi"("error in"=w742, "Precision"="8", "DCPowerInformationByInstrument"=w744) -> ("error out"=w741:errorcluster, "DCPowerInfoArray"=w740:string[][])
        n156 = Insert Into Array(array=w747, index (col)=0 ("disabled index (col)"), new element=w740) -> (w746:string[][])  [unwired: 1 in]
      }
      n157 = Concatenate Strings("Channel Name " ("string")) -> (w631:string)
      n158 = Concatenate Strings("Voltage (V) " ("string")) -> (w633:string)
      n159 = Concatenate Strings("Measure Record delta Time (s) " ("string")) -> (w635:string)
      n160 = Concatenate Strings("Instrument Name " ("string")) -> (w630:string)
      n161 = Concatenate Strings("Instrument Channel Number " ("string")) -> (w632:string)
      n162 = Concatenate Strings("Current Limit (A) " ("string")) -> (w634:string)
      n163 = Build Array(w630, w631, w632, w633, w634, w635) -> (w623:string[])
      n164 = Build Path(base path=w513, name or relative path="DCPOW_Params.csv") -> (appended path=w638:path)
      n165 = Insert Into Array(array=w619, index (col)=0 ("disabled index (col)"), new element=w623) -> (w622:string[][])  [unwired: 1 in]
      n166 = call-poly <vilib>:"Write Delimited Spreadsheet.vi"("file path (dialog if empty)"=w638, "format (%s)"="%s" ("format (%.3f)"), "2D data"=w622, "error in (no error)"=w512, "transpose? (no:F)"=TRUE, "delimiter (\\t)"="," ("delimiter (\\t)")) -> ("error out"=w620:errorcluster)  [unwired: 8 in, 1 out]
      n167 = for {
        shift-right: [w734] -> w600
        shift-left: w620 -> [w734]
        shift-right: [w729] -> w588
        shift-left: w614 -> [w729]
        shift-right: [w730] -> w586
        shift-left: w615 -> [w730]
        shift-right: [w731] -> w584
        shift-left: w616 -> [w731]
        shift-right: [w732] -> w583
        shift-left: w617 -> [w732]
        shift-right: [w733] -> w579
        shift-left: w619 -> [w733]
        tunnel: w618 -> [w728] mode=indexing
        tunnel: [w728] -> w581 mode=indexing
        shift-right: [w697] -> w577
        shift-left: string[][] [] ("DCPowerInfoArray") -> [w703]
        n168 = Unbundle(w728) -> ("instrument handle out"=w727:refnum<k15>, w700:string[], w701:string[], "vertical range"=w722:dbl, "vertical coupling"=w716:T5, "Channel 0 50 ohms?"=w721:bool, "50 ohm vertical range (V)"=w720:dbl, "min record length"=w715:i32, "Actual Sample Rate"=w714:dbl)  [unwired: 1 out]
        n169 = Array Size(array=w700) -> (size(s)=w723:i32)
        n170 = Initialize Array(w722, w723) -> (w719:dbl[])
        n171 = Decimal String To Number(string="8") -> (number=w698:i32)  [unwired: 2 in, 1 out]
        n172 = case shown="True" w721 {
          tunnel: w720 -> [_ w737]
          tunnel: w719 -> [w735 w739]
          tunnel: [w735 w736] -> w718
          frame False {
          }
          frame True {
            n173 = Replace Array Subset(array=w739, new element=w737, index=0) -> (w736:dbl[])
          }
        }
        n174 = Number To Fractional String(number=w714, precision (6)=w698) -> (F-format string=w708:string)  [unwired: 2 in]
        n175 = Number To Decimal String(number=w715) -> (decimal integer string=w709:string)  [unwired: 1 in]
        n176 = Concatenate Strings(w727) -> (w725:string)
        n177 = Number To Fractional String(number=w718, precision (6)=w698) -> (F-format string=w717:string[])  [unwired: 2 in]
        n178 = Number To Decimal String(number=w716) -> (decimal integer string=w710:string)  [unwired: 1 in]
        n179 = Array Size(array=w700) -> (size(s)=w726:i32)
        n180 = Initialize Array(w725, w726) -> (w724:string[])
        n181 = Array Size(array=w700) -> (size(s)=w713:i32)
        n182 = Array Size(array=w700) -> (size(s)=w711:i32)
        n183 = Array Size(array=w700) -> (size(s)=w712:i32)
        n184 = Initialize Array(w710, w713) -> (w707:string[])
        n185 = Initialize Array(w708, w711) -> (w705:string[])
        n186 = Initialize Array(w709, w712) -> (w706:string[])
        n187 = Build Array(w724, w701, w700, w717, w707, w706, w705) -> (w702:string[][])
        n188 = Insert Into Array(array=w703, index (col)=0 ("disabled index (col)"), new element=w702) -> (w697:string[][])  [unwired: 1 in]
      }
      n189 = Build Array("Instrument Name " ("string"), "Channel Name" ("element"), "Instrument Channel Number" ("element"), "Vertical Range (V)" ("element"), "Vertical Coupling" ("element"), "Min Record Length" ("element"), "Actual Sample Rate" ("element")) -> (w604:string[])
      n190 = Insert Into Array(array=w577, index (col)=0 ("disabled index (col)"), new element=w604) -> (w597:string[][])  [unwired: 1 in]
      n191 = Build Path(base path=w513, name or relative path="Oscilloscope_Params.csv") -> (appended path=w602:path)
      n192 = call-poly <vilib>:"Write Delimited Spreadsheet.vi"("file path (dialog if empty)"=w602, "format (%s)"="%s" ("format (%.3f)"), "2D data"=w597, "error in (no error)"=w600, "transpose? (no:F)"=TRUE, "delimiter (\\t)"="," ("delimiter (\\t)")) -> ("error out"=w595:errorcluster)  [unwired: 8 in, 1 out]
      n193 = for {
        shift-right: [w679] -> w593
        shift-left: string[][] [] ("DCPowerInfoArray") -> [w680]
        tunnel: w583 -> [w695] mode=indexing
        shift-right: [w664] -> w569
        shift-left: w595 -> [w671]
        shift-right: [w672] -> w576
        shift-left: w577 -> [w672]
        shift-right: [w673] -> w578
        shift-left: w579 -> [w673]
        shift-right: [w674] -> w580
        shift-left: w581 -> [w674]
        shift-right: [w675] -> w582
        shift-left: w583 -> [w675]
        shift-right: [w676] -> w568
        shift-left: w584 -> [w676]
        shift-right: [w677] -> w585
        shift-left: w586 -> [w677]
        shift-right: [w678] -> w587
        shift-left: w588 -> [w678]
        n194 = Unbundle(w695) -> ("VISA resource name"=w694:refnum<visa-resource-name>, "Frequency (GHz) Output"=w688:dbl, "Power (dBm) Output"=w685:dbl)  [unwired: 2 out]
        n195 = Decimal String To Number(string="8") -> (number=w683:i32)  [unwired: 2 in, 1 out]
        n196 = VISA Write(VISA resource name=w694, write buffer="*IDN?", error in (no error)=w671) -> (VISA resource name out=w690:refnum<visa-resource-name>, return count=w692:u32, error out=w696:errorcluster)
        n197 = Number To Fractional String(number=w685, precision (6)=w683) -> (F-format string=w686:string)  [unwired: 2 in]
        n198 = Add(x=w692, y=u32 10) -> (x+y=w689:u32)
        n199 = Number To Fractional String(number=w688, precision (6)=w683) -> (F-format string=w687:string)  [unwired: 2 in]
        n200 = VISA Read(VISA resource name=w690, byte count=w689, error in (no error)=w696) -> (read buffer=w670:string, error out=w665:errorcluster)  [unwired: 2 out]
        n201 = Search and Replace String(replace all?=TRUE ("replace all? (F)"), input string=w670, search string=",", replace string="_" ("replace string (\"\")"), error in=w665) -> (result string=w667:string, error out=w664:errorcluster)  [unwired: 3 in, 2 out]
        n202 = Build Array(w667, w687, w686) -> (w682:string[])
        n203 = Insert Into Array(array=w680, index (col)=0 ("index (row)"), new element=w682) -> (w679:string[][])  [unwired: 1 in]
      }
      n204 = Build Array("Instrument Name", "Frequency (GHz)" ("element"), "Power (dBm)" ("element")) -> (w589:string[])
      n205 = Build Path(base path=w513, name or relative path="RFSource_Params.csv") -> (appended path=w574:path)
      n206 = Insert Into Array(array=w593, index (col)=0 ("disabled index (col)"), new element=w589) -> (w570:string[][])  [unwired: 1 in]
      n207 = call-poly <vilib>:"Write Delimited Spreadsheet.vi"("file path (dialog if empty)"=w574, "format (%s)"="%s" ("format (%.3f)"), "2D data"=w570, "error in (no error)"=w569, "transpose? (no:F)"=TRUE, "delimiter (\\t)"="," ("delimiter (\\t)")) -> ("error out"=w549:errorcluster)  [unwired: 8 in, 1 out]
      n208 = Strip Path(path=w513) -> (name=w567:string)  [unwired: 1 out]
      n209 = Unbundle(w568) -> ("DUT"=w566:string, "Ion (ex Kr)"=w565:string, "Board Number"=w564:string, "Effective LET"=w563:string, "Test Type"=w562:T15)  [unwired: 1 out]
      n210 = case shown="\"Single Event Latchup\", Default" w562 {
        tunnel: ["Single Event Latchup (SEL)" "Single Event Transient (SET)"] -> w561
        frame "Single Event Latchup", Default {
        }
        frame "Single Event Transient" {
        }
      }
      n211 = Build Array("Run Number" ("name"), "DUT" ("element"), "Ion" ("element"), "Board Number" ("element"), "Effective LET" ("element"), "Test Type" ("element")) -> (w560:string[])
      n212 = Build Array(w567, w566, w565, w564, w563, w561) -> (w559:string[])
      n213 = Build Array(w560, w559) -> (w548:string[][])
      n214 = Build Path(base path=w513, name or relative path="RunData_Params.csv") -> (appended path=w554:path)
      n215 = call-poly <vilib>:"Write Delimited Spreadsheet.vi"("file path (dialog if empty)"=w554, "format (%s)"="%s" ("format (%.3f)"), "2D data"=w548, "error in (no error)"=w549, "transpose? (no:F)"=TRUE, "delimiter (\\t)"="," ("delimiter (\\t)")) -> ()  [unwired: 8 in, 2 out]
      n216 = List Folder(path=w513, pattern="*NULL.txt") -> (path out=w532:path, filenames=w533:string[], error out=w534:errorcluster)  [unwired: 2 in, 1 out]
      n217 = for {
        tunnel: [w649] -> w544
        tunnel: w532 -> [w649]
        tunnel: w533 -> [w651] mode=indexing
        shift-right: [w652] -> w535
        shift-left: w534 -> [w653]
        n218 = Build Path(base path=w649, name or relative path=w651) -> (appended path=w650:path)
        n219 = Delete(path (use dialog)=w650, error in=w653) -> (error out=w652:errorcluster)  [unwired: 3 in, 2 out]
      }
      n220 = Get Date/Time String(date format (0)=enum16{"short", "long", "abbreviated"}."short", seconds (now)=w514, want seconds? (F)=TRUE) -> (date string=w538:string, time string=w537:string)
      n221 = Concatenate Strings(w538, "_" ("string"), w537) -> (w539:string)
      n222 = Strip Path(path=w544) -> (name=w530:string)  [unwired: 1 out]
      n223 = Build Path(base path=w544, name or relative path="BeginRecordTimeStamp.txt") -> (appended path=w545:path)
      n224 = Concatenate Strings(w530, "_DCPOWER_COPYFOLDER" ("name or relative path")) -> (w531:string)
      n225 = Open/Create/Replace File(file path (use dialog)=w545, error in=w535, operation (0:open)=T14."open or create", access (0:read/write)=enum16{"read/write", "read-only", "write-only"}."read/write") -> (refnum out=w540:refnum<file>, error out=w536:errorcluster)  [unwired: 2 in, 1 out]
      n226 = Build Path(base path=w544, name or relative path=w531) -> (appended path=w524:path)
      n227 = Write to Text File(file (use dialog)=w540, text=w539, error in=w536) -> (refnum out=w542:refnum<file>, error out=w541:errorcluster)  [unwired: 1 in, 1 out]
      n228 = Close File(refnum=w542, error in=w541) -> (error out=w543:errorcluster)  [unwired: 1 out]
      n229 = Create Folder(path (use dialog)=w524, error in=w543) -> (created path=w528:path, error out=w525:errorcluster)  [unwired: 1 in, 1 out]
      n230 = List Folder(path=w544, error in=w525) -> (path out=w526:path, filenames=w527:string[], error out=w529:errorcluster)  [unwired: 2 in, 1 out]
      n231 = for {
        tunnel: w526 -> [w659]
        tunnel: w527 -> [w658] mode=indexing
        tunnel: w528 -> [w654]
        shift-right: [w661] -> w515
        shift-left: w529 -> [w655]
        tunnel: [w654] -> _
        n232 = Build Path(base path=w659, name or relative path=w658) -> (appended path=w656:path)
        n233 = Build Path(base path=w654, name or relative path=w658) -> (appended path=w657:path)
        n234 = Copy(8:w655, 9:TRUE ("overwrite (F)"), 10:w657, 11:w656) -> (0:w661:errorcluster)  [unwired: 1 in, 2 out]
      }
    }
  }
  "DCPowerInformationClusterArray_Output" <- w35
  "VISAPowerInfoInputOutput" <- w37
  "Run Data SubPanel Output" <- w39
  "Data Was Collected?" <- w32
  "DCPowerInfoArray" <- w31
  "OscilloscopeInfoArray" <- w2
  "RFSourceInfoArray" <- w20
  "RF Subpanel Output" <- w41
  "error out" <- w7
  "Oscilloscope Info Array" <- w1
